vi "Send Notifier.vi"(8 "Error In":errorcluster, 11 "notifier in":refnum<notifier>) -> (0 "Error Out":errorcluster, 3 "notifier out":refnum<notifier>)   [LabVIEW 2019, in "Error Notifier.lvlib"]
uses:
  Error Notifier.lvlib
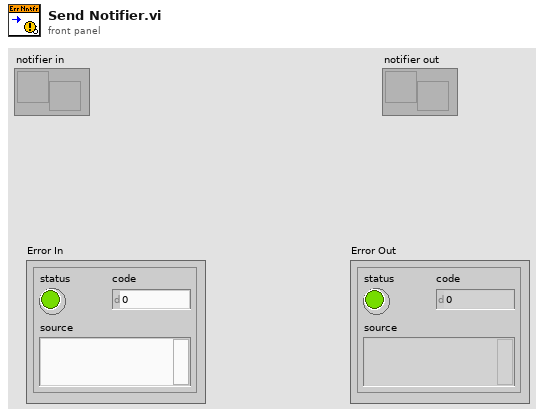
[diagram p1: front panel]
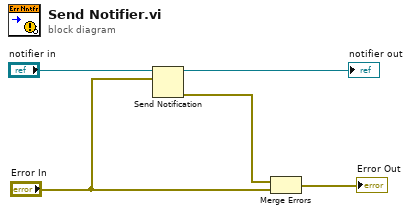
[diagram p0: block diagram]
diagram:
  n1 = Send Notification(notification="Error In", notifier="notifier in") -> (notifier out=→"notifier out":refnum<notifier>, error out=w1:errorcluster)  [unwired: 1 in]
  n2 = Merge Errors(w1, "Error In") -> (→"Error Out":errorcluster)
